vi "Write Msg Attributes.vi"(10 "Msg Attributes":refnum<data-value>, 11 "Actor in":refnum<class "Actor.lvclass">) -> (3 "Actor out":refnum<class "Actor.lvclass">)   [LabVIEW 2020, in "jettl.lvlib" / "Actor.lvclass"]
uses:
  Actor.lvclass
  Relation.ctl
  jettl.lvlib
  Teller.ctl
  Msg Attributes.ctl
  Msg Input/Msg Input.lvclass
  Msg Output/Msg Output.lvclass
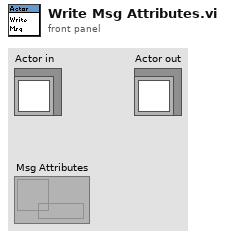
[diagram p1: front panel]
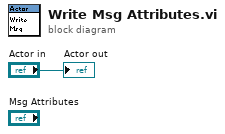
[diagram p0: block diagram]
diagram:
  "Actor out" <- "Actor in"
